vi "WLM Wait for server.vi"(8 "error in (no error)":errorcluster, 10 "loop delay (ms) (100)":u32=100, 11 "Timeout (ms) (10000)":u32=10000) -> (0 "error out":errorcluster)   [LabVIEW 2012]
doc: "Waits for a server to be active, and returns either when one is active or after timing out."
uses:
  <vilib>/Utility/error.llb/DialogType.ctl
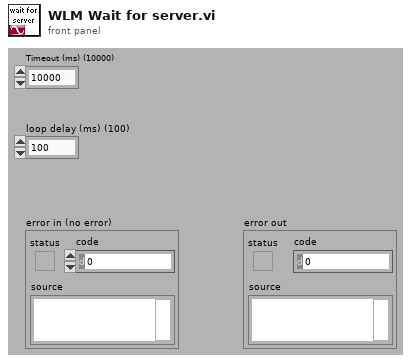
[diagram p1: front panel]
types:
  T1 = typedef "DialogType.ctl" = u16
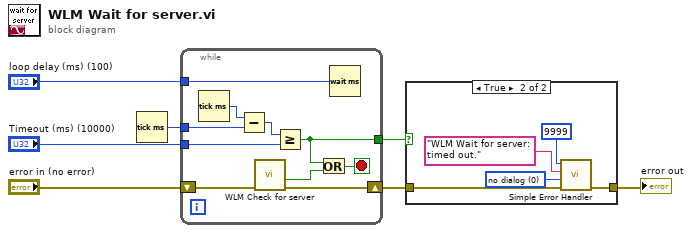
[diagram p0: block diagram]
diagram:
  n1 = Tick Count (ms)() -> (millisecond timer value=w6:u32)
  n2 = while {
    shift-right: [w17] -> w2
    shift-left: "error in (no error)" -> [w16]
    tunnel: w6 -> [w14]
    tunnel: "Timeout (ms) (10000)" -> [w12]
    tunnel: [w9] -> w3
    tunnel: "loop delay (ms) (100)" -> [w8]
    stop <- w10 stop-if-true
    n3 = Tick Count (ms)() -> (millisecond timer value=w15:u32)
    n4 = Subtract(x=w15, y=w14) -> (x-y=w13:u32)
    n5 = call "WLM Check for server.vi"("error in (no error)"=w16) -> ("error out"=w17:errorcluster, "WLM server running?"=w11:bool)  [unwired: 9 out]
    n6 = Greater Or Equal?(x=w13, y=w12) -> (x >= y?=w9:bool)
    n7 = Or(x=w9, y=w11) -> (x .or. y?=w10:bool)
    n8 = Wait (ms)(milliseconds to wait=w8) -> ()  [unwired: 1 out]
  }
  n9 = case shown="True" w3 {
    tunnel: w2 -> [w18 w23]
    tunnel: [w18 w19] -> w1
    frame False {
    }
    frame True {
      w21 = T1 0 items=["no dialog", "OK message", "continue or stop message", "OK message + warnings", "continue/stop + warnings"] ("type of dialog (OK msg:1)")
      n10 = call <vilib>:"Simple Error Handler.vi"("error code (no error:0)"=9999, "error source (\" \")"="WLM Wait for server: timed out." ("error source (\" \")"), "type of dialog (OK msg:1)"=w21, "error in (no error)"=w23) -> ("error out"=w19:errorcluster)  [unwired: 5 out]
    }
  }
  "error out" <- w1
